vi "Status Input.vi"(0 "VISA resource name":refnum<visa-resource-name>, 5 "Input Group (0:Inputs 1-4)":u16(ring) items=["Inputs 1-4", "Inputs 5-8"], 9 "Input (1)":dbl=1.0 min=1.0 max=8.0 step=1.0, 11 "error in (no error)":errorcluster) -> (4 "VISA resource name out":refnum<visa-resource-name>, 6 "Input Group":u16(ring) items=["2.5V Diode", "7.5V Diode", "250 Ohm Platinum", "500 Ohm Platinum", "5K Ohm Platinum", "Cernox"], 8 "Input Off/On":bool, 10 "Input Curve":u16(ring) items=["None", "DT-470", "DT-500", "CTI Diode", "Empty Standard Diode", "Empty Standard Diode", "PT-100", "PT-1000", "Empty Standard Platinum", "Empty Standard Platinum", "Unused", "Unused", "Unused", "Unused", "Unused", "Unused", "Unused", "Unused", "Unused", "Unused", "Unused", "User Curve 1", "User Curve 2", "User Curve 3", "User Curve 4", "User Curve 5", "User Curve 6", "User Curve 7", "User Curve 8"], 15 "error out":errorcluster)   [LabVIEW 2017, in "Lake Shore Cryotronics 218.lvlib"]
doc: "This VI reads the status of the following parameters of the 218 inputs:\n\nSensor type for each input group.\nIndividual inputs on and off.\nIndicates Curve for individual inputs."
uses:
  Lake Shore Cryotronics 218.lvlib
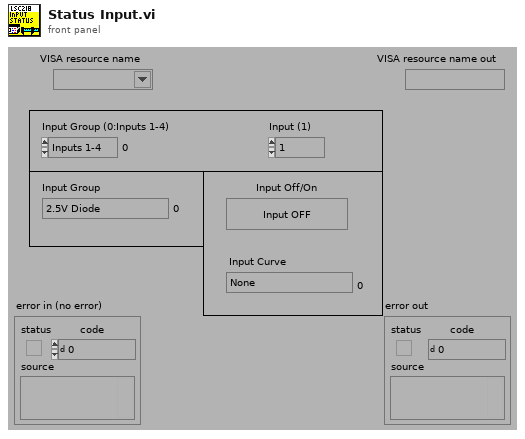
[diagram p1: front panel]
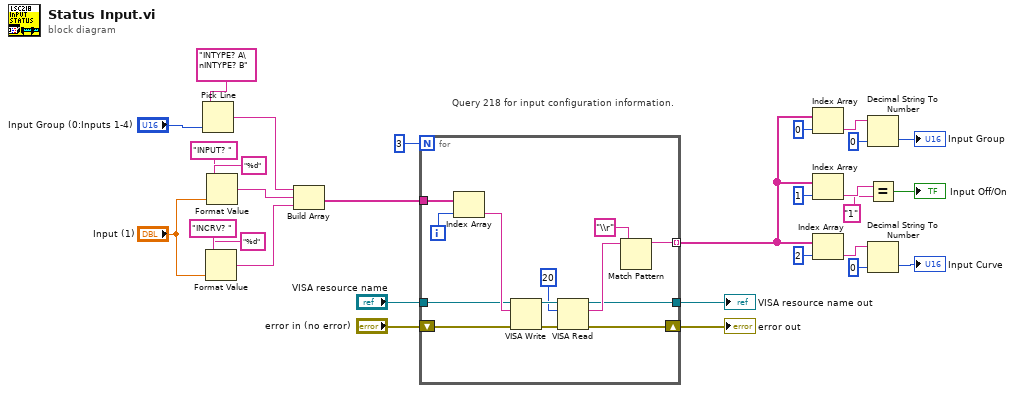
[diagram p0: block diagram]
diagram:
  # "Query 218 for input configuration information."
  n1 = Pick Line(multi-line string="INTYPE? A\nINTYPE? B", line index="Input Group (0:Inputs 1-4)") -> (output string=w21:string)  [unwired: 1 in]
  n2 = Format Value(string ("")="INCRV? ", format string="%d", value (0)="Input (1)") -> (output string=w18:string)
  n3 = Format Value(string ("")="INPUT? ", format string="%d", value (0)="Input (1)") -> (output string=w19:string)
  n4 = Build Array(w21, w19, w18) -> (w22:string[])
  n5 = for {
    N: 3 -> [_]
    tunnel: [w38] -> w15 mode=indexing
    shift-right: [w35] -> w4
    shift-left: "error in (no error)" -> [w36]
    tunnel: [w34] -> w5
    tunnel: w22 -> [w32]
    tunnel: "VISA resource name" -> [w31]
    i -> [w37]
    n6 = Index Array(array=w32, index=w37) -> (element=w33:string)
    n7 = VISA Write(VISA resource name=w31, write buffer=w33, error in (no error)=w36) -> (VISA resource name out=w42:refnum<visa-resource-name>, error out=w41:errorcluster)  [unwired: 1 out]
    n8 = VISA Read(VISA resource name=w42, byte count=20, error in (no error)=w41) -> (VISA resource name out=w34:refnum<visa-resource-name>, read buffer=w39:string, error out=w35:errorcluster)  [unwired: 1 out]
    n9 = Match Pattern(string=w39, regular expression="\\r") -> (before substring=w38:string)  [unwired: 1 in, 3 out]
  }
  "error out" <- w4
  "VISA resource name out" <- w5
  n10 = Index Array(array=w15, index=0) -> (element=w14:string)
  n11 = Index Array(array=w15, index=1) -> (element=w12:string)
  n12 = Index Array(array=w15, index=2) -> (element=w9:string)
  n13 = Decimal String To Number(string=w14, default (0L)=u16 0) -> (number=→"Input Group":u16)  [unwired: 1 in, 1 out]
  n14 = Equal?(x=w12, y="1") -> (x = y?=→"Input Off/On":bool)
  n15 = Decimal String To Number(string=w9, default (0L)=u16 0) -> (number=→"Input Curve":u16)  [unwired: 1 in, 1 out]
